vi "Anything to Variant Database.vi"(8 "Error In":errorcluster, 11 "Type of Anything":variant) -> (0 "Error Out":errorcluster, 3 "Variant Database":variant)   [LabVIEW 2020]
doc: "This VI was created for use with the Read/Write Cluster VIs. It reads all the keys and their values from the specified section and puts them in two string arrays.\n\nFreeware from Moore Good Ideas, www.mooregoodideas.com. Do not remove this line."
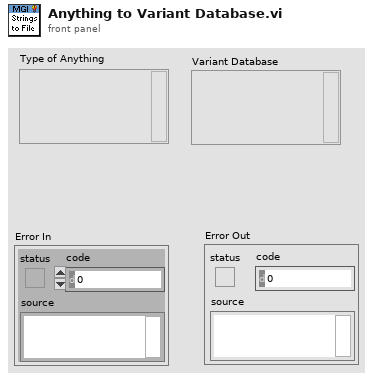
[diagram p1: front panel]
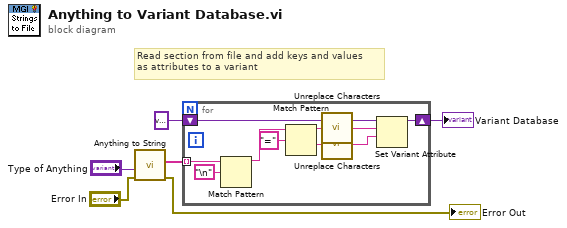
[diagram p0: block diagram]
diagram:
  # "Read section from file and add keys and values\nas attributes to a variant"
  n1 = call "Anything to String.vi"("Error In"="Error In", "Anything"="Type of Anything") -> ("Error Out"=→"Error Out":errorcluster, "Strings[]"=w3:string[])  [unwired: 7 in, 1 out]
  n2 = for {
    shift-right: [w14] -> w5
    shift-left: variant ("variant") -> [w15]
    tunnel: w3 -> [w8] mode=indexing
    n3 = Match Pattern(string=w8, regular expression="\n") -> (before substring=w9:string)  [unwired: 1 in, 3 out]
    n4 = Match Pattern(string=w9, regular expression="=") -> (before substring=w13:string, after substring=w12:string)  [unwired: 1 in, 2 out]
    n5 = call "Unreplace Characters.vi"("String In"=w13) -> ("String Out"=w11:string)  [unwired: 1 in]
    n6 = call "Unreplace Characters.vi"("String In"=w12) -> ("String Out"=w10:string)  [unwired: 1 in]
    n7 = Set Variant Attribute(Variant=w15, name=w11, value=w10) -> (Variant out=w14:variant)  [unwired: 1 in, 2 out]
  }
  "Variant Database" <- w5
